vi "OE1022D_Configure Ref Phase.vi"(7 "OE1022D_Configure Ref Phase":T1={"Sweep Mode"=0, "Start Frequency(Hz)"=1000.0, "Stop Frequency(Hz)"=0.001, "Linear Step Frequency(Hz)"=1000.0, "Log Step Percent(%)"=10.0, "Step Time(ms)"=1000, "Sweep Run Mode"=0, "Internal Frequency(Hz)"=1000.0, "Phase  (degree)"=0.0, "External Ref Trigger"=0, "Reference Source"=0, "Channel"=1} {"Channel" items=["A"=1, "B"=2]; "Reference Source" items=["External", "Internal", "Internal Sweep", "Channel-A"]; "External Ref Trigger" items=["TTL Rising Edge", "TTL Falling Edge", "Sine Zero Crossing"]; "Phase  (degree)" min=-180.0 max=180.0 format="%#.2g"; "Internal Frequency(Hz)" min=0.001 max=102000.0 format="%#.3f"; "Sweep Run Mode" items=["Stop", "Singal", "Loop"]; "Step Time(ms)" min=1 max=100000; "Log Step Percent(%)" min=0.0 max=100.0 format="%#.2g"; "Linear Step Frequency(Hz)" min=0.001 max=102000.0 format="%#.3f"; "Stop Frequency(Hz)" min=0.001 max=102000.0 format="%#.3f"; "Start Frequency(Hz)" min=0.001 max=102000.0 format="%#.3f"; "Sweep Mode" items=["Linear", "Log"]}, 8 "Error in (no error)":errorcluster caption="error out（no error）", 9 "Remote Mode":u16(ring) items=["USB", "RS232", "GPIB"], 11 "VISA resource name":refnum<visa-resource-name>) -> (0 "Error out":errorcluster caption="error out", 1 "Output String":string, 3 "VISA resource  out":refnum<visa-resource-name>)   [LabVIEW 2019]
panel:
  out "字符串":string
  # "PS: When you set the \"Channel A\" option in the reference source, only \"Channel B\" can be selected. \nIf \"Channel A\" is selected, the setting will not respond."
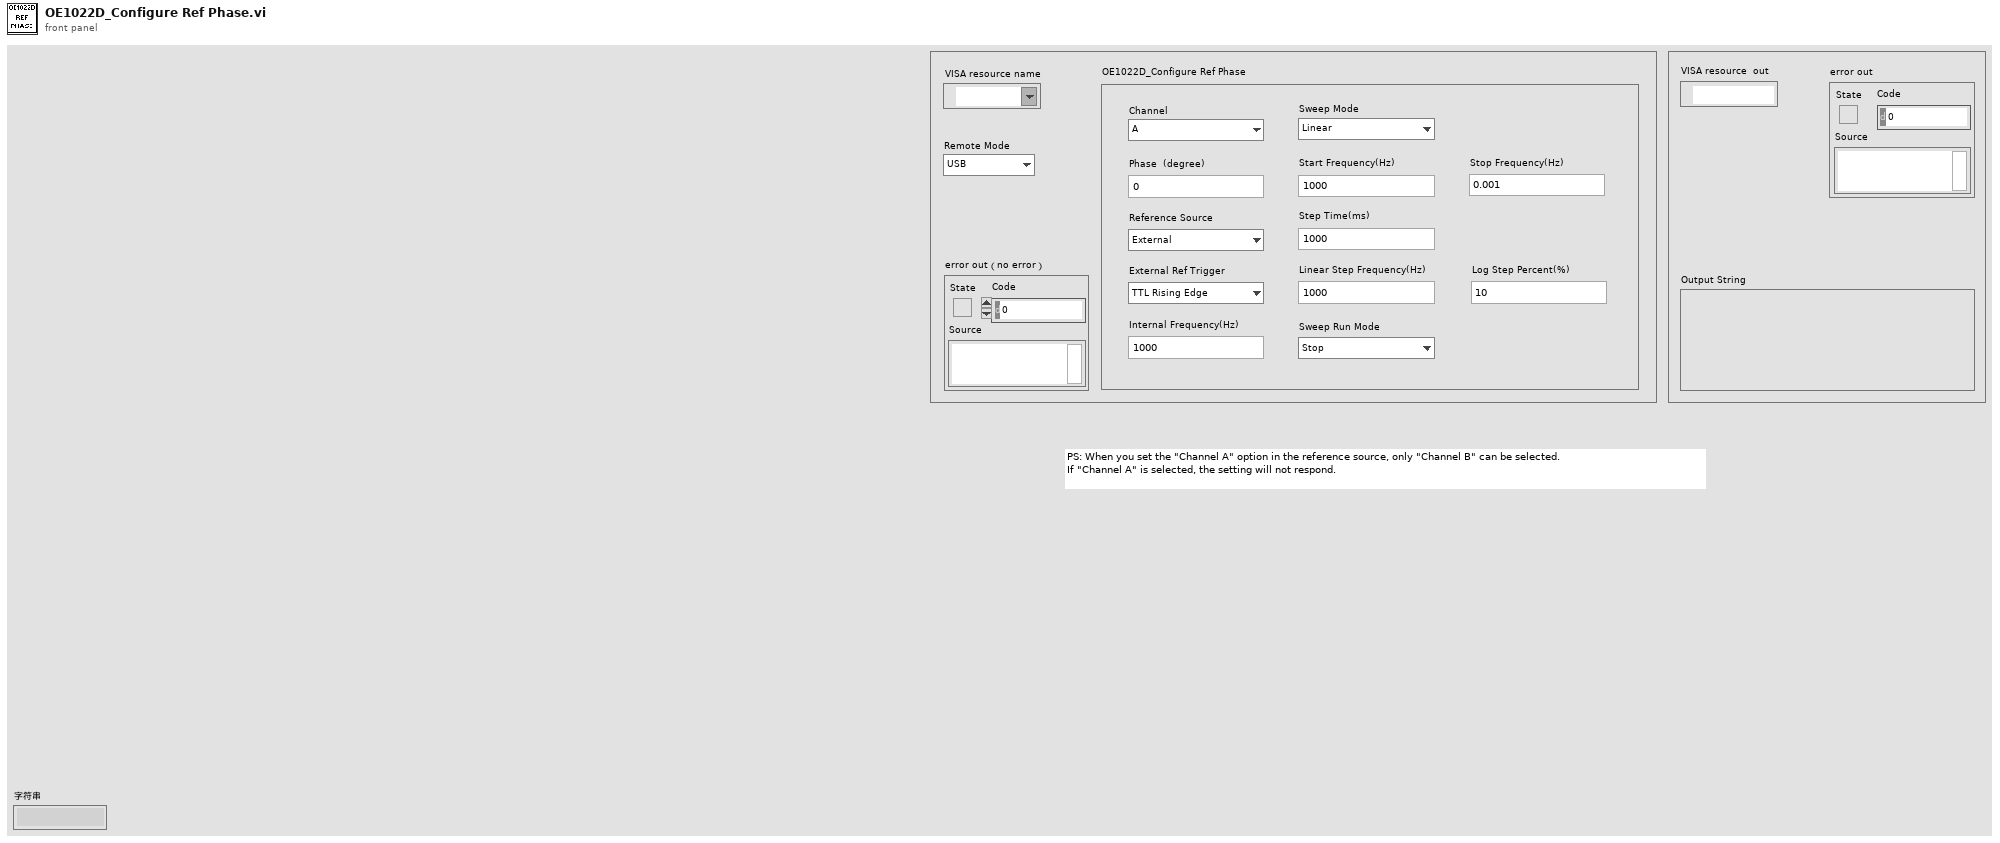
[diagram p1: front panel]
types:
  T1 = cluster{"Sweep Mode":u16, "Start Frequency(Hz)":dbl, "Stop Frequency(Hz)":dbl, "Linear Step Frequency(Hz)":dbl, "Log Step Percent(%)":dbl, "Step Time(ms)":u32, "Sweep Run Mode":u16, "Internal Frequency(Hz)":dbl, "Phase  (degree)":dbl, "External Ref Trigger":u16, "Reference Source":u16, "Channel":u16}
  T2 = enum16{"ISRC", "IGND", "ICPL", "ILIN", "PHAS", "FMOD", "RSLP", "FREQ", "SWPT", "SLLM", "SULM", "SSLL", "SSLG", "STLM", "SWRM", "IRNG", "SENS", "RMOD", "OFLT", "OFSL", "SYNC", "DMOD", "HARM", "DARB", "SWVT", "SLVL", "SVLL", "SVUL", "SVSL", "SVSG", "SVTM", "SVRM", "RALL", "SNAP", "OUTP", "OAUX", "COUT", "CAUX", "COFP", "CEXP", "FPOP", "OEXP", "*IDN", "*RST", "OVLD", "INOV", "GNOV", "*PLL", "SSET", "RSET", "AGAN", "APHS", "ARSV", "ASCL", "EQCD", "EQCS", "SPED", "SRAT", "SLEN", "SSLE", "STRG", "SPRM", "STRD", "PAUS", "REST", "SPTS", "TRCA", "TEMP", "RSTU", "IHNZ", "DEQU", "SADD", "ARNG", "CSPE", "ISRCD", "IGNDD", "ICPLD", "ILIND", "PHASD", "FMODD", "RSLPD", "FREQD", "SWPTD", "SLLMD", "SULMD", "SSLLD", "SSLGD", "STLMD", "SWRMD", "SENSD", "RMODD", "OFLTD", "OFSLD", "SYNCD", "HARMD", "EQCDD", "EQCSD", "SNAPD", "OUTPD", "SWVTD", "SLVLD", "SVLLD", "SVULD", "SVSLD", "SVSGD", "SVTMD", "SVRMD", "SVDCD", "ARSVD", "AGAND", "APHSD", "ASCLD", "FPOPD", "CAUXD", "OEXPD", "SPEDD", "SRATD", "SLEND", "SSLED", "STRGD", "SPRMD", "STRDD", "PAUSD", "RESTD", "SPTSD", "TRCAD", "*IDND", "*RSTD", "INOVD", "GNOVD", "*PLLD", "SSETD", "RSETD"}
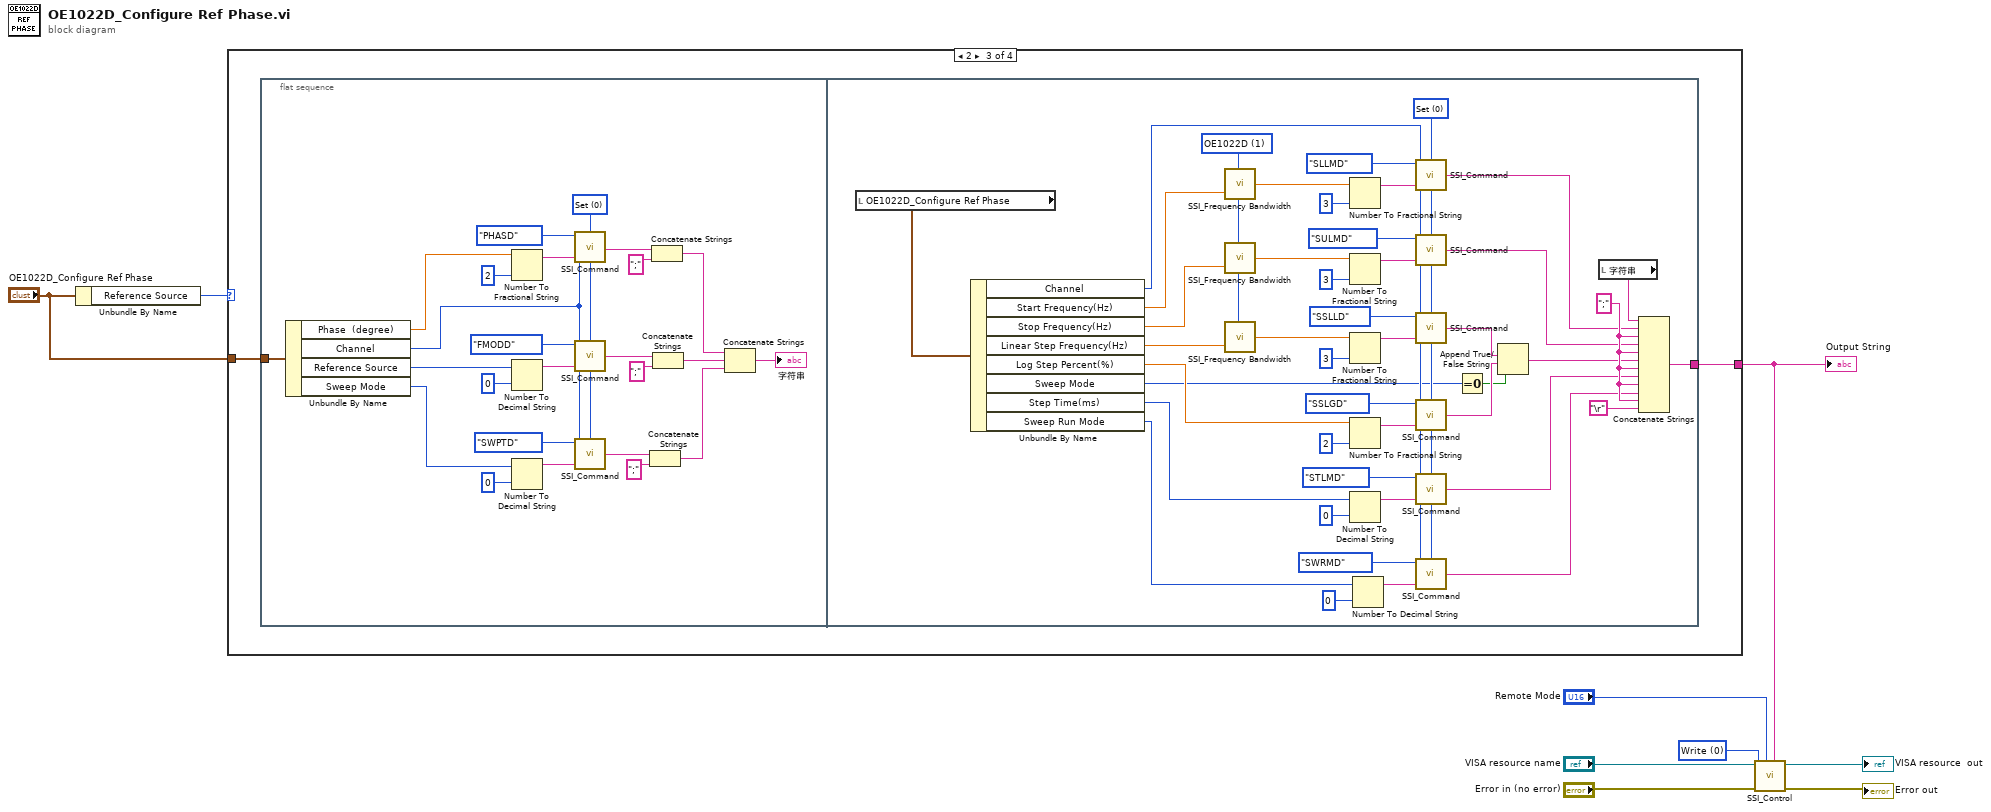
[diagram p0: block diagram]
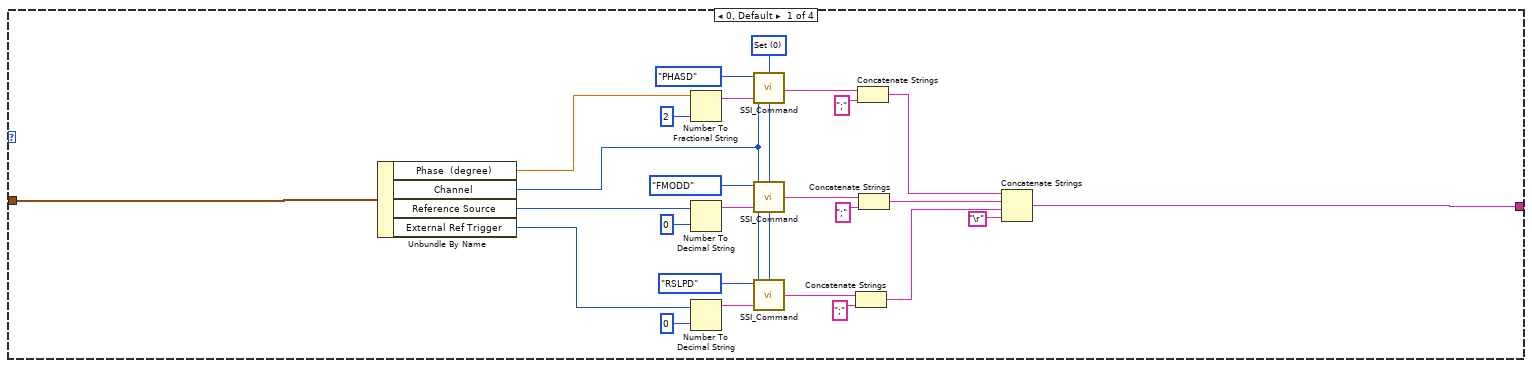
[diagram p2: hidden frame]
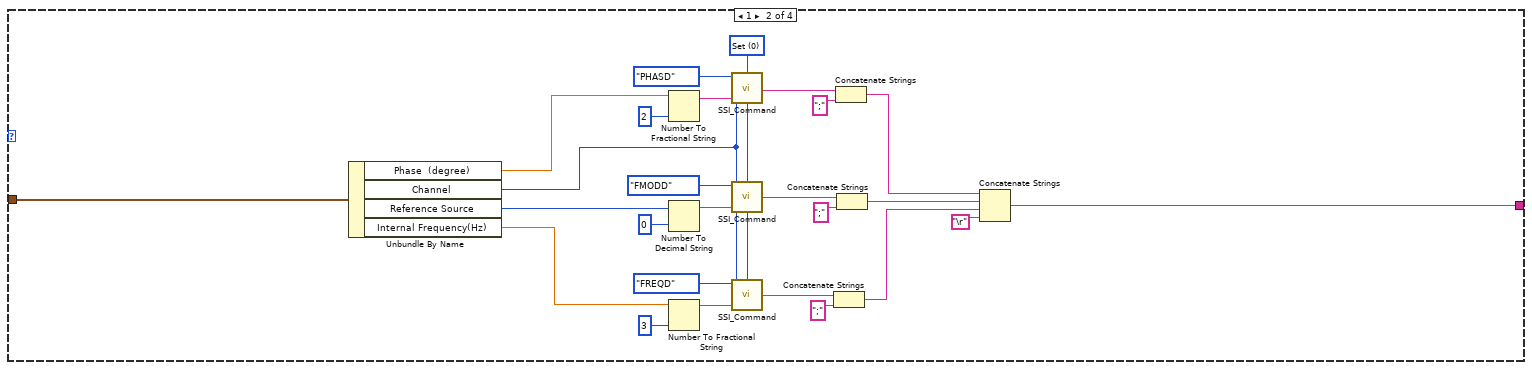
[diagram p3: hidden frame]
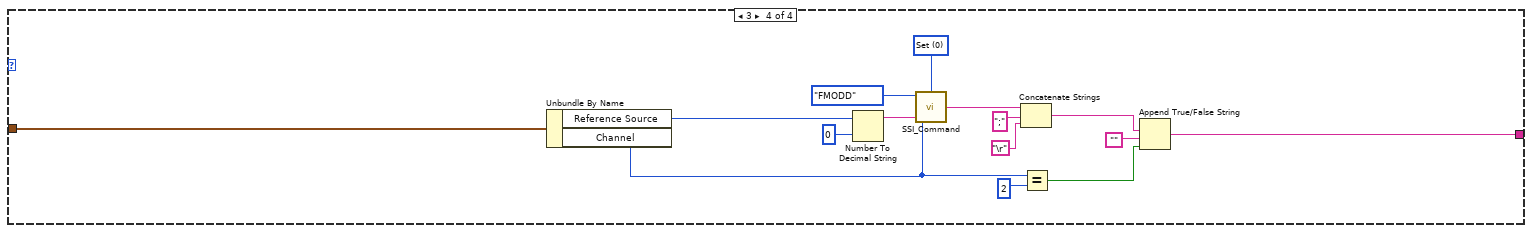
[diagram p4: hidden frame]
diagram:
  w7 = u16 0 items=["Write", "Read"] ("Control")
  n1 = Unbundle By Name("OE1022D_Configure Ref Phase") -> ("Reference Source"=w3:u16)
  n2 = case shown="2" w3 {
    tunnel: "OE1022D_Configure Ref Phase" -> [w17 w38 w63 w140]
    tunnel: [w11 w37 w62 w136] -> w1
    frame 0, Default {
      w16 = u16 0 items=["Set", "Query"] ("Opera")
      n3 = Unbundle By Name(w17) -> ("Phase  (degree)"=w19:dbl, "Channel"=w18:u16, "Reference Source"=w15:u16, "External Ref Trigger"=w20:u16)
      n4 = Number To Fractional String(number=w19, precision (6)=i16 2 ("精度(6)")) -> (F-format string=w34:string)  [unwired: 2 in]
      n5 = Number To Decimal String(number=w15, width (-)=i16 0 ("精度(6)")) -> (decimal integer string=w31:string)
      n6 = Number To Decimal String(number=w20, width (-)=i16 0 ("精度(6)")) -> (decimal integer string=w28:string)
      n7 = call "SSI_Command.vi"("Opera"=w16, "Paramter"=w34, "channel"=w18, "Command Type"=T2."PHASD") -> ("Output string"=w21:string)
      n8 = call "SSI_Command.vi"("Opera"=w16, "Paramter"=w31, "channel"=w18, "Command Type"=T2."FMODD") -> ("Output string"=w23:string)
      n9 = call "SSI_Command.vi"("Opera"=w16, "Paramter"=w28, "channel"=w18, "Command Type"=T2."RSLPD") -> ("Output string"=w26:string)
      n10 = Concatenate Strings(w26, ";" ("替换字符串(\"\")")) -> (w12:string)
      n11 = Concatenate Strings(w21, ";" ("替换字符串(\"\")")) -> (w14:string)
      n12 = Concatenate Strings(w23, ";" ("替换字符串(\"\")")) -> (w13:string)
      n13 = Concatenate Strings(w14, w13, w12, "\r") -> (w11:string)
    }
    frame 1 {
      w43 = u16 0 items=["Set", "Query"] ("Opera")
      n14 = Unbundle By Name(w38) -> ("Phase  (degree)"=w45:dbl, "Channel"=w44:u16, "Reference Source"=w42:u16, "Internal Frequency(Hz)"=w46:dbl)
      n15 = Number To Fractional String(number=w45, precision (6)=i16 2 ("精度(6)")) -> (F-format string=w60:string)  [unwired: 2 in]
      n16 = Number To Decimal String(number=w42, width (-)=i16 0 ("精度(6)")) -> (decimal integer string=w57:string)
      n17 = Number To Fractional String(number=w46, precision (6)=i16 3 ("精度(6)")) -> (F-format string=w54:string)  [unwired: 2 in]
      n18 = call "SSI_Command.vi"("Opera"=w43, "Paramter"=w60, "channel"=w44, "Command Type"=T2."PHASD") -> ("Output string"=w47:string)
      n19 = call "SSI_Command.vi"("Opera"=w43, "Paramter"=w57, "channel"=w44, "Command Type"=T2."FMODD") -> ("Output string"=w49:string)
      n20 = call "SSI_Command.vi"("Opera"=w43, "Paramter"=w54, "channel"=w44, "Command Type"=T2."FREQD") -> ("Output string"=w52:string)
      n21 = Concatenate Strings(w52, ";" ("替换字符串(\"\")")) -> (w39:string)
      n22 = Concatenate Strings(w47, ";" ("替换字符串(\"\")")) -> (w41:string)
      n23 = Concatenate Strings(w49, ";" ("替换字符串(\"\")")) -> (w40:string)
      n24 = Concatenate Strings(w41, w40, w39, "\r") -> (w37:string)
    }
    frame 2 {
      n25 = flat-sequence {
        tunnel: w63 -> [w65]
        tunnel: [w92] -> w62
        frame #0 {
          w70 = u16 0 items=["Set", "Query"] ("Opera")
          n26 = Unbundle By Name(w65) -> ("Phase  (degree)"=w72:dbl, "Channel"=w71:u16, "Reference Source"=w69:u16, "Sweep Mode"=w73:u16)
          n27 = Number To Fractional String(number=w72, precision (6)=i16 2 ("精度(6)")) -> (F-format string=w87:string)  [unwired: 2 in]
          n28 = Number To Decimal String(number=w69, width (-)=i16 0 ("精度(6)")) -> (decimal integer string=w84:string)
          n29 = Number To Decimal String(number=w73, width (-)=i16 0 ("精度(6)")) -> (decimal integer string=w81:string)
          n30 = call "SSI_Command.vi"("Opera"=w70, "Paramter"=w87, "channel"=w71, "Command Type"=T2."PHASD") -> ("Output string"=w74:string)
          n31 = call "SSI_Command.vi"("Opera"=w70, "Paramter"=w84, "channel"=w71, "Command Type"=T2."FMODD") -> ("Output string"=w76:string)
          n32 = call "SSI_Command.vi"("Opera"=w70, "Paramter"=w81, "channel"=w71, "Command Type"=T2."SWPTD") -> ("Output string"=w79:string)
          n33 = Concatenate Strings(w79, ";" ("替换字符串(\"\")")) -> (w66:string)
          n34 = Concatenate Strings(w74, ";" ("替换字符串(\"\")")) -> (w68:string)
          n35 = Concatenate Strings(w76, ";" ("替换字符串(\"\")")) -> (w67:string)
          n36 = Concatenate Strings(w68, w67, w66) -> (→"字符串":string)
        }
        frame #1 {
          w132 = u16 1 items=["OE1022", "OE1022D", "OE1201", "OE1311", "OE1351", "OE1301", "OE2031-10M", "OE2041-30M", "OE2041-60M"] ("Instrument Mode")
          w131 = ";"
          w121 = u16 0 items=["Set", "Query"] ("Opera")
          n37 = local read "OE1022D_Configure Ref Phase"() -> (w93:T1)
          n38 = Unbundle By Name(w93) -> ("Channel"=w95:u16, "Start Frequency(Hz)"=w99:dbl, "Stop Frequency(Hz)"=w98:dbl, "Linear Step Frequency(Hz)"=w97:dbl, "Log Step Percent(%)"=w94:dbl, "Sweep Mode"=w91:u16, "Step Time(ms)"=w90:u32, "Sweep Run Mode"=w89:u16)
          n39 = call "SSI_Frequency Bandwidth.vi"("Frequency"=w99, "Instrument Mode"=w132) -> ("Output"=w102:dbl)  [unwired: 1 in]
          n40 = call "SSI_Frequency Bandwidth.vi"("Frequency"=w98, "Instrument Mode"=w132) -> ("Output"=w101:dbl)  [unwired: 1 in]
          n41 = call "SSI_Frequency Bandwidth.vi"("Frequency"=w97, "Instrument Mode"=w132) -> ("Output"=w100:dbl)  [unwired: 1 in]
          n42 = Number To Fractional String(number=w102, precision (6)=i16 3 ("精度(6)")) -> (F-format string=w116:string)  [unwired: 2 in]
          n43 = Number To Fractional String(number=w101, precision (6)=i16 3 ("精度(6)")) -> (F-format string=w113:string)  [unwired: 2 in]
          n44 = Number To Fractional String(number=w100, precision (6)=i16 3 ("精度(6)")) -> (F-format string=w110:string)  [unwired: 2 in]
          n45 = Number To Fractional String(number=w94, precision (6)=i16 2 ("精度(6)")) -> (F-format string=w107:string)  [unwired: 2 in]
          n46 = Number To Decimal String(number=w90, width (-)=i16 0 ("精度(6)")) -> (decimal integer string=w104:string)
          n47 = Number To Decimal String(number=w89, width (-)=i16 0 ("精度(6)")) -> (decimal integer string=w119:string)
          n48 = call "SSI_Command.vi"("Opera"=w121, "Paramter"=w116, "channel"=w95, "Command Type"=T2."SLLMD") -> ("Output string"=w125:string)
          n49 = call "SSI_Command.vi"("Opera"=w121, "Paramter"=w113, "channel"=w95, "Command Type"=T2."SULMD") -> ("Output string"=w126:string)
          n50 = call "SSI_Command.vi"("Opera"=w121, "Paramter"=w110, "channel"=w95, "Command Type"=T2."SSLLD") -> ("Output string"=w123:string)
          n51 = call "SSI_Command.vi"("Opera"=w121, "Paramter"=w107, "channel"=w95, "Command Type"=T2."SSLGD") -> ("Output string"=w124:string)
          n52 = call "SSI_Command.vi"("Opera"=w121, "Paramter"=w104, "channel"=w95, "Command Type"=T2."STLMD") -> ("Output string"=w128:string)
          n53 = call "SSI_Command.vi"("Opera"=w121, "Paramter"=w119, "channel"=w95, "Command Type"=T2."SWRMD") -> ("Output string"=w129:string)
          n54 = Equal To 0?(x=w91) -> (x = 0?=w122:bool)
          n55 = Append True/False String(1:w122, 2:w124, 3:w123) -> (0:w127:string)  [unwired: 1 in]
          n56 = local read "字符串"() -> (w96:string)
          n57 = Concatenate Strings(w96, w125, w131, w126, w131, w127, w131, w128, w131, w129, w131, "\r") -> (w92:string)
        }
      }
    }
    frame 3 {
      w142 = u16 0 items=["Set", "Query"] ("Opera")
      n58 = Unbundle By Name(w140) -> ("Reference Source"=w141:u16, "Channel"=w133:u16)
      n59 = Number To Decimal String(number=w141, width (-)=i16 0 ("精度(6)")) -> (decimal integer string=w146:string)
      n60 = call "SSI_Command.vi"("Opera"=w142, "Paramter"=w146, "channel"=w133, "Command Type"=T2."FMODD") -> ("Output string"=w143:string)
      n61 = Concatenate Strings(w143, ";" ("替换字符串(\"\")"), "\r") -> (w134:string)
      n62 = Equal?(x=w133, y=u16 2) -> (x = y?=w138:bool)
      n63 = Append True/False String(1:w138, 2:"", 3:w134) -> (0:w136:string)  [unwired: 1 in]
    }
  }
  "Output String" <- w1
  n64 = call "SSI_Control.vi"("Write Buffer"=w1, "Remote Mode"="Remote Mode", "Error in (no error)"="Error in (no error)", "Control"=w7, "VISA resource name"="VISA resource name") -> ("Error out"=→"Error out":errorcluster, "VISA resource  out"=→"VISA resource  out":refnum<visa-resource-name>)  [unwired: 3 in, 2 out]
